vi "Make unpersistent.vi"(8 "error in (no error)":errorcluster, 11 "PS Control Persistence Actor in":refnum<class "PS Control Persistence Actor.lvclass">) -> (0 "error out":errorcluster, 3 "PS Control Persistence Actor out":refnum<class "PS Control Persistence Actor.lvclass">)   [LabVIEW 2025, in "PS Control Persistence.lvlib" / "PS Control Persistence Actor.lvclass"]
doc: "Author: Scott Hannahs <sth@magnet.fsu.edu>\n\nThis software is licensed for use under the “MIT License\"\nCopyright (c) 2025 Scott Hannahs, sth@sth@magnet.sthnet.net\n\nPermission is hereby granted, free of charge, to any person obtaining a copy of this software and associated documentation files (the \"Software\"), to deal in the Software without restriction, including without limitation the rights to use, copy, modify, merge, publish, distribute, sublicense, and/or sell copies of the Software, and to permit persons to whom the Software is furnished to do so, subject to the following conditions: The above copyright notice and this permission notice shall be included in all copies or substantial portions of the Software.\n\nTHE SOFTWARE IS PROVIDED \"AS IS\", WITHOUT WARRANTY OF ANY KIND, EXPRESS OR IMPLIED, INCLUDING BUT NOT LIMITED TO THE WARRANTIES OF MERCHANTABILITY, FITNESS FOR A PARTICULAR PURPOSE AND NONINFRINGEMENT. IN NO EVENT SHALL THE AUTHORS OR COPYRIGHT HOLDERS BE LIABLE FOR ANY CLAIM, DAMAGES OR OTHER LIABILITY, WHETHER IN AN ACTION OF CONTRACT, TORT OR OTHERWISE, ARISING FROM, OUT OF OR IN CONNECTION WITH THE SOFTWARE OR THE USE OR OTHER DEALINGS IN THE SOFTWARE."
uses:
  PS Control Persistence Actor.lvclass
  PS Driver/PS Driver with Persistence.lvclass
  PS Control Actor.lvclass/PS Control Actor.ctl
  PS Control Actor.lvclass
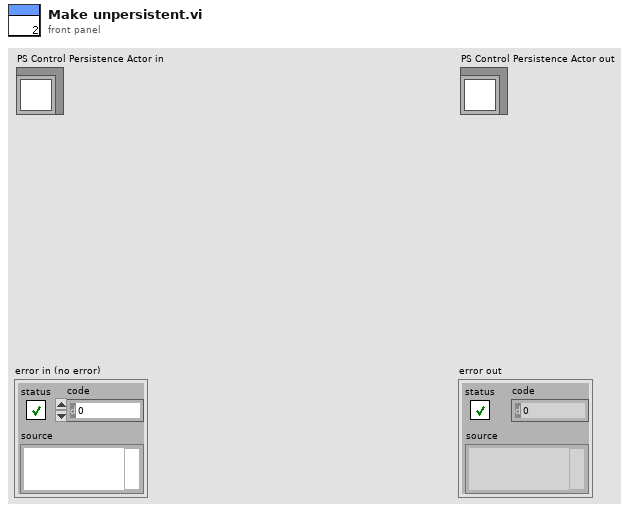
[diagram p1: front panel]
types:
  T1 = enum8{"Enabled", "Disabled", "Disabled and Grayed Out"}
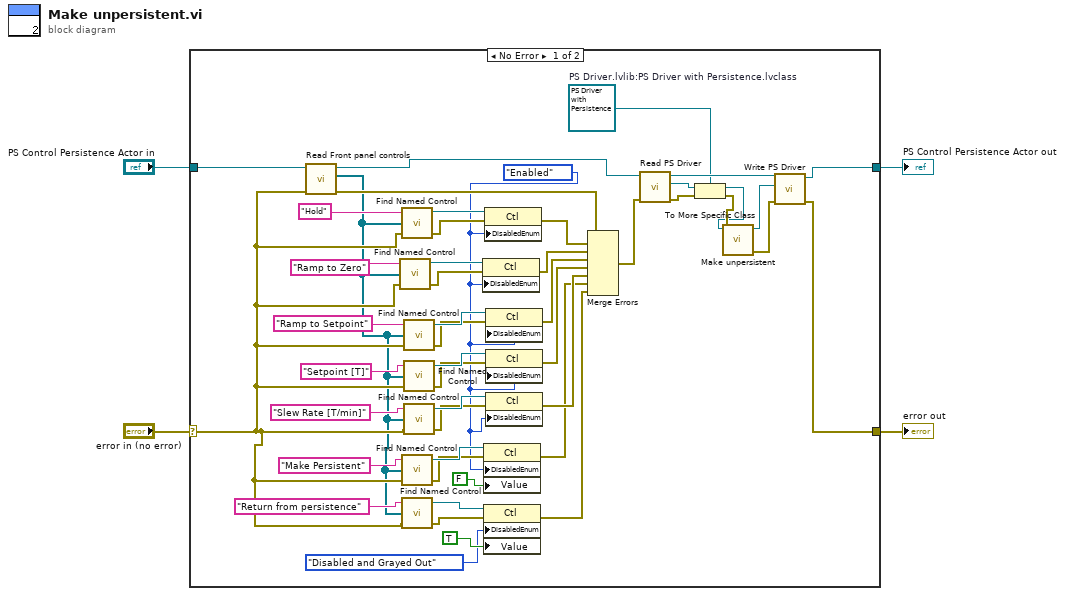
[diagram p0: block diagram]
diagram:
  n1 = case shown="No Error" "error in (no error)" {
    selector: "error in (no error)" -> [w10 w54]
    tunnel: [w27 w54] -> w4
    tunnel: [w28 w53] -> w3
    tunnel: "PS Control Persistence Actor in" -> [w40 w53]
    frame No Error {
      w23 = refnum<class "PS Driver with Persistence.lvclass"> refnum  # PS Driver.lvlib:PS Driver with Persistence.lvclass
      w5 = T1."Enabled" ("Disabled")
      n2 = call "Read Front panel controls.vi"("error in (no error)"=w10, "PS Control Actor in"=w40) -> ("error out"=w39:errorcluster, "Front panel controls"=w9:refnum<vi>[], "PS Control Actor out"=w30:refnum<class "PS Control Persistence Actor.lvclass">)  [unwired: 7 in]
      n3 = call "Find Named Control.vi"("error in"=w10, "All Controls"=w9, "Control Name"="Ramp to Zero") -> ("error out"=w48:errorcluster, "Ctl Refnum"=w49:refnum<vi>)  [unwired: 1 out]
      n4 = call "Find Named Control.vi"("error in"=w10, "All Controls"=w9, "Control Name"="Hold") -> ("error out"=w51:errorcluster, "Ctl Refnum"=w52:refnum<vi>)  [unwired: 1 out]
      n5 = call "Find Named Control.vi"("error in"=w10, "All Controls"=w9, "Control Name"="Make Persistent") -> ("error out"=w17:errorcluster, "Ctl Refnum"=w18:refnum<vi>)  [unwired: 1 out]
      n6 = call "Find Named Control.vi"("error in"=w10, "All Controls"=w9, "Control Name"="Return from persistence") -> ("error out"=w15:errorcluster, "Ctl Refnum"=w16:refnum<vi>)  [unwired: 1 out]
      n7 = call "Find Named Control.vi"("error in"=w10, "All Controls"=w9, "Control Name"="Ramp to Setpoint") -> ("error out"=w43:errorcluster, "Ctl Refnum"=w44:refnum<vi>)  [unwired: 1 out]
      n8 = call "Find Named Control.vi"("error in"=w10, "All Controls"=w9, "Control Name"="Setpoint [T]") -> ("error out"=w37:errorcluster, "Ctl Refnum"=w38:refnum<vi>)  [unwired: 1 out]
      n9 = call "Find Named Control.vi"("error in"=w10, "All Controls"=w9, "Control Name"="Slew Rate [T/min]") -> ("error out"=w35:errorcluster, "Ctl Refnum"=w36:refnum<vi>)  [unwired: 1 out]
      n10 = property class="Ctl"(reference=w49, error in=w48, "DisabledEnum"=w5) -> (error out=w45:errorcluster)  [unwired: 1 out]
      n11 = property class="Ctl"(reference=w18, error in=w17, "DisabledEnum"=w5, "Value"=FALSE) -> (error out=w8:errorcluster)  [unwired: 1 out]
      n12 = property class="Ctl"(reference=w16, error in=w15, "DisabledEnum"=T1."Disabled and Grayed Out" ("Disabled"), "Value"=TRUE) -> (error out=w7:errorcluster)  [unwired: 1 out]
      n13 = property class="Ctl"(reference=w52, error in=w51, "DisabledEnum"=w5) -> (error out=w46:errorcluster)  [unwired: 1 out]
      n14 = property class="Ctl"(reference=w44, error in=w43, "DisabledEnum"=w5) -> (error out=w41:errorcluster)  [unwired: 1 out]
      n15 = property class="Ctl"(reference=w38, error in=w37, "DisabledEnum"=w5) -> (error out=w32:errorcluster)  [unwired: 1 out]
      n16 = property class="Ctl"(reference=w36, error in=w35, "DisabledEnum"=w5) -> (error out=w31:errorcluster)  [unwired: 1 out]
      n17 = Merge Errors(w39, w46, w45, w41, w32, w31, w8, w7) -> (w26:errorcluster)
      n18 = call-dynamic "Read PS Driver.vi"("error in (no error)"=w26, "PS Control Persistence Actor in"=w30) -> ("error out"=w25:errorcluster, "PS Driver.lvlib:PS Driver.lvclass"=w24:refnum<class "PS Driver.lvclass">, "PS Control Persistence Actor out"=w29:refnum<class "PS Control Persistence Actor.lvclass">)  [unwired: 7 in]
      n19 = To More Specific Class(target class=w23, reference=w24, error in=w25) -> (specific class reference=w19:refnum<class "PS Driver with Persistence.lvclass">, error out=w20:errorcluster)
      n20 = call-dynamic "Make unpersistent.vi"("error in (no error)"=w20, "PS Driver with Persistence in"=w19) -> ("error out"=w22:errorcluster, "PS Driver with Persistence out"=w21:refnum<class "PS Driver with Persistence.lvclass">)  [unwired: 8 in]
      n21 = call-dynamic "Write PS Driver.vi"("error in (no error)"=w22, "PS Driver.lvlib:PS Driver.lvclass"=w21, "PS Control Persistence Actor in"=w29) -> ("error out"=w27:errorcluster, "PS Control Persistence Actor out"=w28:refnum<class "PS Control Persistence Actor.lvclass">)  [unwired: 7 in]
    }
    frame Error {
    }
  }
  "error out" <- w4
  "PS Control Persistence Actor out" <- w3
